vi "InverseA (SubVI).vi"(1 "PtsFrame1":T2[](array[typedef])) -> (0 "inverseA":T1)   [LabVIEW 2021]
uses:
  ctrOWLMarker.ctl
  <vilib>/Analysis/Matrix/Datatypes/RealMatrix.ctl
  <vilib>/Analysis/_algsub.llb/Real PseudoInverse Matrix.vi
  <vilib>/Analysis/Matrix/Numeric/Conversions/Array To Matrix - RA2.vi
  <vilib>/Analysis/Matrix/NI_Matrix.lvlib
  <vilib>/Analysis/NI_AALPro.lvlib
panel:
  out "A":T1
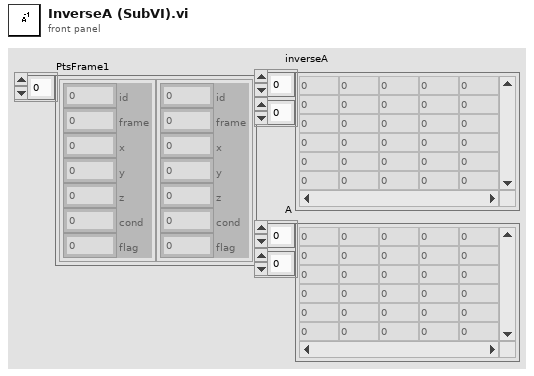
[diagram p1: front panel]
types:
  T1 = typedef "NI_Matrix.lvlib/RealMatrix.ctl" = dbl[][]
  T2 = typedef "ctrOWLMarker.ctl" = cluster{"id":i32, "frame":i32, "x":sgl, "y":sgl, "z":sgl, "cond":sgl, "flag":u32}
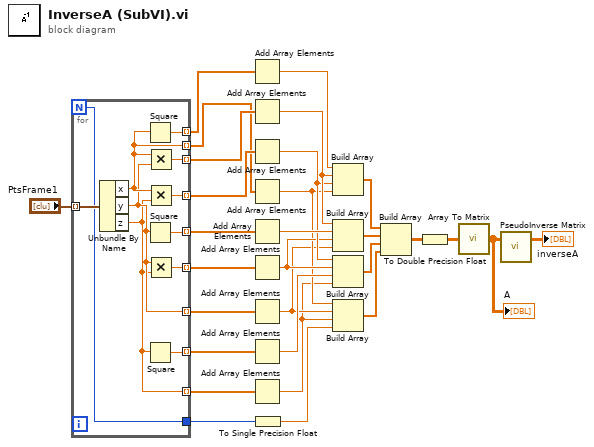
[diagram p0: block diagram]
diagram:
  n1 = for {
    N -> [w30]
    tunnel: "PtsFrame1" -> [w40] mode=indexing
    tunnel: [w39] -> w24 mode=indexing
    tunnel: [w38] -> w25 mode=indexing
    tunnel: [w37] -> w26 mode=indexing
    tunnel: [w36] -> w27 mode=indexing
    tunnel: [w35] -> w28 mode=indexing
    tunnel: [w34] -> w29 mode=indexing
    tunnel: [w33] -> w23 mode=indexing
    tunnel: [w32] -> w22 mode=indexing
    tunnel: [w31] -> w21 mode=indexing
    tunnel: [w30] -> w10
    n2 = Unbundle By Name(w40) -> ("x"=w33:sgl, "y"=w32:sgl, "z"=w31:sgl)
    n3 = Square(x=w33) -> (x^2=w39:sgl)
    n4 = Square(x=w32) -> (x^2=w38:sgl)
    n5 = Square(x=w31) -> (x^2=w37:sgl)
    n6 = Multiply(x=w33, y=w32) -> (x*y=w36:sgl)
    n7 = Multiply(x=w33, y=w31) -> (x*y=w34:sgl)
    n8 = Multiply(x=w32, y=w31) -> (x*y=w35:sgl)
  }
  n9 = Add Array Elements(numeric array=w24) -> (sum=w20:sgl)
  n10 = Add Array Elements(numeric array=w27) -> (sum=w19:sgl)
  n11 = Add Array Elements(numeric array=w29) -> (sum=w17:sgl)
  n12 = Add Array Elements(numeric array=w23) -> (sum=w14:sgl)
  n13 = Add Array Elements(numeric array=w25) -> (sum=w18:sgl)
  n14 = Add Array Elements(numeric array=w28) -> (sum=w16:sgl)
  n15 = Add Array Elements(numeric array=w22) -> (sum=w13:sgl)
  n16 = Add Array Elements(numeric array=w26) -> (sum=w15:sgl)
  n17 = Add Array Elements(numeric array=w21) -> (sum=w12:sgl)
  n18 = To Single Precision Float(number=w10) -> (single precision float=w9:sgl)
  n19 = Build Array(w20, w19, w17, w14) -> (w8:sgl[])
  n20 = Build Array(w19, w18, w16, w13) -> (w7:sgl[])
  n21 = Build Array(w17, w16, w15, w12) -> (w6:sgl[])
  n22 = Build Array(w14, w13, w12, w9) -> (w5:sgl[])
  n23 = Build Array(w8, w7, w6, w5) -> (w4:sgl[][])
  n24 = To Double Precision Float(number=w4) -> (double precision float=w3:dbl[][])
  n25 = call-poly <vilib>:"Array To Matrix.vi"("Real 2D Array"=w3) -> ("Real Matrix"=w2:T1)
  "A" <- w2
  n26 = call-poly <vilib>:"PseudoInverse Matrix.vi"("Input Matrix"=w2) -> ("PseudoInverse Matrix"=→"inverseA":T1)  [unwired: 1 in, 1 out]
